vi "Create Queue Connection.vi"(5 "Connection.LocalQueue":refnum<class "Connection.LocalQueue.lvclass">, 8 "error in (no error)":errorcluster, 9 "Queue Name":string, 10 "Outbound":refnum<queue>, 11 "Inbound":refnum<queue>) -> (0 "error out":errorcluster, 3 "Connection.LocalQueue":refnum<class "Connection.LocalQueue.lvclass">)   [LabVIEW 2013, in "Connection.Queue_GOSPL.lvlib" / "Connection.LocalQueue.lvclass"]
uses:
  Connection.LocalQueue.lvclass
  Connection.LocalQueue.lvclass/Connection.LocalQueue.ctl
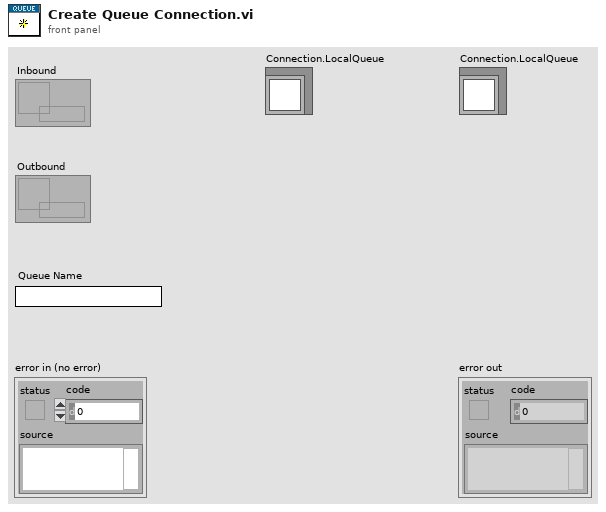
[diagram p1: front panel]
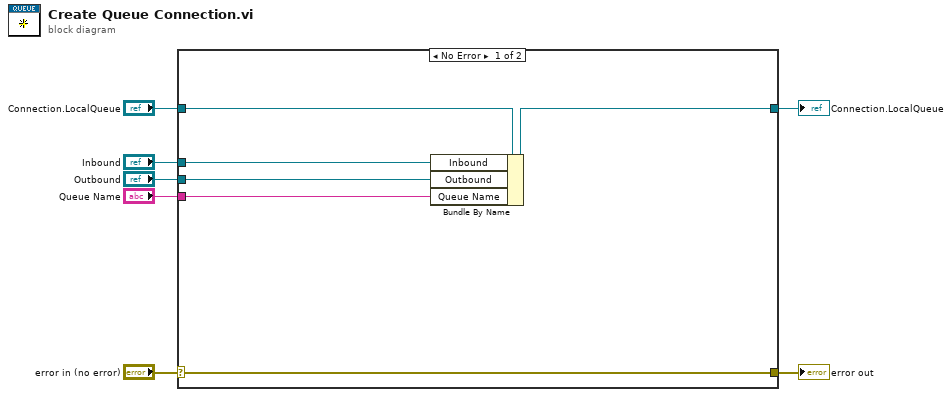
[diagram p0: block diagram]
diagram:
  n1 = case shown="No Error" "error in (no error)" {
    selector: "error in (no error)" -> [w12 w15]
    tunnel: [w12 w15] -> w6
    tunnel: [w11 w14] -> w4
    tunnel: "Connection.LocalQueue" -> [w13 w14]
    tunnel: "Inbound" -> [w10 _]
    tunnel: "Queue Name" -> [w9 _]
    tunnel: "Outbound" -> [w8 _]
    frame No Error {
      n2 = Bundle By Name(cluster=w13, "Inbound"=w10, "Outbound"=w8, "Queue Name"=w9) -> (w11:refnum<class "Connection.LocalQueue.lvclass">)
    }
    frame Error {
    }
  }
  "error out" <- w6
  "Connection.LocalQueue" <- w4
